vi "Get Thread Parameters.vi"(11 "Transceiver Thread in":refnum<class "Plugin Thread.lvclass">) -> (2 "Thread Parameters":refnum<class "Thread Parameters.lvclass">, 3 "Transceiver Thread out":refnum<class "Plugin Thread.lvclass">)   [LabVIEW 2017, in "DSF Core.lvlib" / "Plugin Thread.lvclass"]
uses:
  Plugin Thread.lvclass
  Thread Parameters/Thread Parameters.lvclass
  Plugin Thread.lvclass/Plugin Thread.ctl
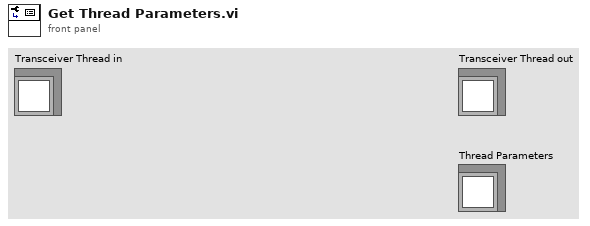
[diagram p1: front panel]
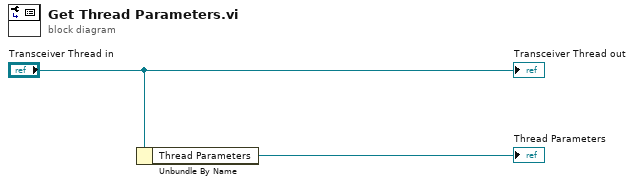
[diagram p0: block diagram]
diagram:
  n1 = Unbundle By Name("Transceiver Thread in") -> ("Thread Parameters"=→"Thread Parameters":refnum<class "Thread Parameters.lvclass">)
  "Transceiver Thread out" <- "Transceiver Thread in"
